vi "add_noise.vi"(8 "error in (no error)":errorcluster, 11 "Image in":refnum<class "Image.lvclass">) -> (0 "error out":errorcluster, 3 "Image out":refnum<class "Image.lvclass">)   [LabVIEW 2010, in "Image.lvclass"]
uses:
  Image.lvclass
  ErrorController/ErrorController/class_data.vi
  ErrorController/ErrorController/ErrorController.lvclass
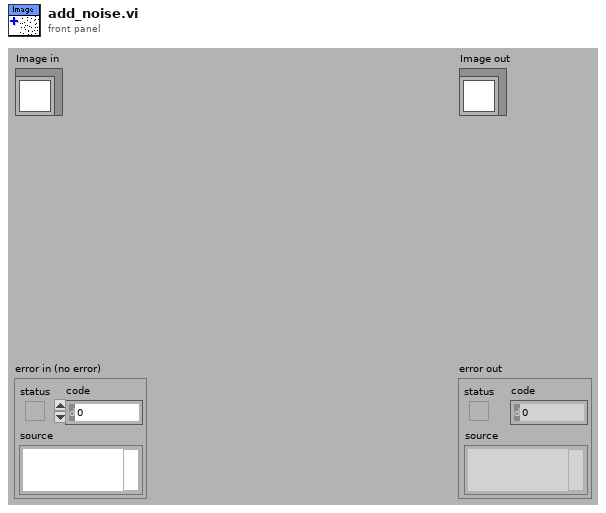
[diagram p1: front panel]
types:
  T1 = typedef "Image Type" = u32
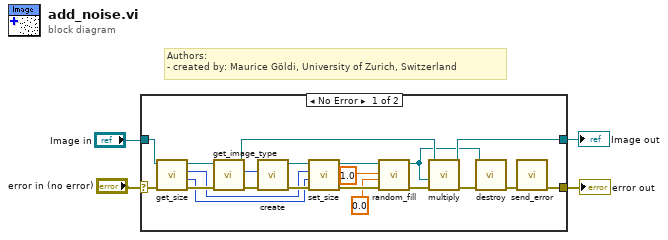
[diagram p0: block diagram]
diagram:
  # "Authors: \n- created by: Maurice Göldi, University of Zurich, Switzerland"
  n1 = case shown="No Error" "error in (no error)" {
    selector: "error in (no error)" -> [w23 w27]
    tunnel: [w5 w27] -> w3
    tunnel: [w10 w26] -> w1
    tunnel: "Image in" -> [w21 w26]
    frame No Error {
      n2 = call-dynamic "get_size.vi"("error in (no error)"=w23, "Image in"=w21) -> ("error out"=w22:errorcluster, "y resolution"=w14:i32, "x resolution"=w15:i32, "Image out"=w20:refnum<class "Image.lvclass">)  [unwired: 6 out]
      n3 = call-dynamic "get_image_type.vi"("error in (no error)"=w22, "Image.lvclass in"=w20) -> ("error out"=w25:errorcluster, "Image Type"=w24:T1, "Image.lvclass out"=w11:refnum<class "Image.lvclass">)  [unwired: 7 out]
      n4 = call "create.vi"("error in (no error)"=w25, "Image Type"=w24) -> ("error out"=w19:errorcluster, "Image out"=w17:refnum<class "Image.lvclass">)  [unwired: 2 in, 6 out]
      n5 = call-dynamic "set_size.vi"("error in (no error)"=w19, "y"=w14, "x"=w15, "Image in"=w17) -> ("error out"=w18:errorcluster, "Image out"=w16:refnum<class "Image.lvclass">)  [unwired: 6 out]
      n6 = call-dynamic "random_fill.vi"("error in (no error)"=w18, "minimum value"=0.0, "maximum value"=1.0, "Image in"=w16) -> ("error out"=w8:errorcluster, "Image out"=w7:refnum<class "Image.lvclass">)  [unwired: 6 out]
      n7 = call-dynamic "multiply.vi"("error in (no error)"=w8, "factor image"=w7, "Image in"=w11) -> ("error out"=w9:errorcluster, "Image out"=w10:refnum<class "Image.lvclass">)  [unwired: 1 in, 6 out]
      n8 = call-dynamic "destroy.vi"("error in (no error)"=w9, "Image in"=w7) -> ("error out"=w6:errorcluster)  [unwired: 9 out]
      n9 = call "send_error.vi"("error in (no error)"=w6) -> ("error out"=w5:errorcluster)  [unwired: 10 in]
    }
    frame Error {
    }
  }
  "error out" <- w3
  "Image out" <- w1
